vi "Test_Crop_ARGB.vi"(8 "error in (no error)":errorcluster, 11 "Test Case In":refnum<class "Image.lvclass">) -> (0 "error out":errorcluster, 3 "Test Case Out":refnum<class "Image.lvclass">)   [LabVIEW 2020, in "g_ar_toolkit.test.lvlib" / "Image.lvclass"]
uses:
  Image.lvclass
  Image.lvclass/Image.ctl
  g_ar_toolkit.image/g_ar_toolkit.image.lvlib
  g_ar_toolkit.image/Image Size (Fixed).ctl
  g_ar_toolkit.image/CreateEmptyImageARGB.vi
  g_ar_toolkit.image/Image Point (Fixed).ctl
  4993e8ee-a06a-463a-9684-69129f64d5ce.vi
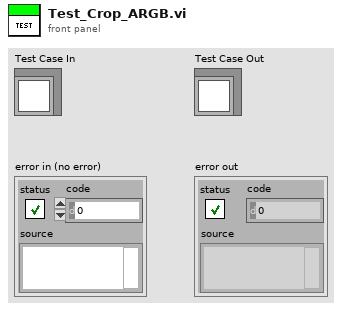
[diagram p1: front panel]
types:
  T1 = typedef "g_ar_toolkit.image.lvlib/Image Point (Fixed).ctl" = cluster{"x":i32, "y":i32}
  T2 = typedef "g_ar_toolkit.image.lvlib/Image Size (Fixed).ctl" = cluster{"Width":u16, "Height":u16}
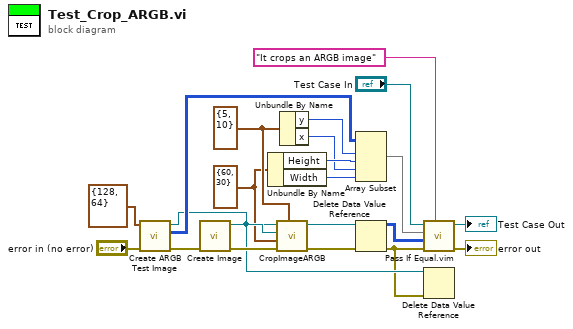
[diagram p0: block diagram]
diagram:
  w10 = T1 {"x"=5, "y"=10} ("Origin (Default: 0,0)")
  w9 = T2 {"Width"=60, "Height"=30} ("Cropped Size")
  n1 = call "Create ARGB Test Image.vi"("error in (no error)"="error in (no error)", "Preallocated Image Size"=T2 {"Width"=128, "Height"=64} ("Preallocated Image Size (Default - 0,0)")) -> ("error out"=w12:errorcluster, "24-bit pixmap"=w11:u32[][], "Data Value Reference out"=w2:refnum<data-value>)  [unwired: 7 in]
  n2 = call-poly "Create Image.vi"("error in (no error)"=w12) -> ("error out"=w16:errorcluster, "New ARGB Image"=w14:refnum<data-value>)  [unwired: 9 in]
  n3 = Unbundle By Name(w9) -> ("Height"=w8:u16, "Width"=w5:u16)
  n4 = call "CropImageARGB.vi"("Origin (Default: 0,0)"=w10, "error in (no error)"=w16, "Cropped Size"=w9, "ARGB Image Destination"=w14, "ARGB Image Source"=w2) -> ("error out"=w18:errorcluster, "ARGB Image Destination (duplicate)"=w3:refnum<data-value>)  [unwired: 5 in]
  n5 = Unbundle By Name(w10) -> ("y"=w7:i32, "x"=w6:i32)
  n6 = Array Subset(array=w11, index (row)=w7, length (row)=w8, index (col)=w6, length (col)=w5) -> (w4:u32[][])
  n7 = Delete Data Value Reference(data value reference=w3, error in=w18) -> (data value=w15:u32[][], error out=w1:errorcluster)
  n8 = call "Pass If Equal.vim"("Description"="It crops an ARGB image", "error in (no error)"=w1, "Actual"=w15, "Expected"=w4, "LUnit Test Case In"="Test Case In") -> ("error out"=→"error out":errorcluster, "LUnit Test Case Out"=→"Test Case Out":refnum<class "Image.lvclass">)  [unwired: 5 in]
  n9 = Delete Data Value Reference(data value reference=w2, error in=w1) -> ()  [unwired: 2 out]
